vi "fit elliptical orbit to many magnetometer readings.vi"(6 "minimums":T2={"a"=0.0, "b"=-300.0, "theta_axis"=-7.0, "dPhi"=-0.1, "BrV"=-10000.0, "bob tilt"=-0.3, "phi0"=-7.0, "phi_dot"=-1.0, "x0"=-10.0, "y0"=-10.0, "z0"=-200.0}, 7 "maximums":T2={"a"=300.0, "b"=300.0, "theta_axis"=7.0, "dPhi"=0.1, "BrV"=10000.0, "bob tilt"=0.3, "phi0"=7.0, "phi_dot"=1.0, "x0"=10.0, "y0"=10.0, "z0"=200.0}, 8 "t0":fxp<+,48,48>, 9 "omega":dbl, 10 "magnetometer readings":T3[](array[typedef]), 11 "initial parameters":T2) -> (0 "fit field":dbl[](array[numeric]), 1 "measured field":dbl[](array[numeric]), 2 "predicted location":dbl[][](array[numeric]), 3 "fit parameters":T2, 4 "initial field prediction":dbl[](array[numeric]), 5 "initial predicted location":dbl[][](array[numeric]))   [LabVIEW 2017]
uses:
  typedefs/orbit parameters full.ctl
  typedefs/magnetomter reading set.ctl
  typedefs/orbit magnetic field data.ctl
  <vilib>/gmath/NumericalOptimization/Nonlinear Curve Fit TRDL bound.vi
  <vilib>/gmath/NI_Gmath.lvlib
panel:
  out "number of function calls":i32
  out "residue":dbl
  out "initial deriv nan":bool
  out "initial guess nan":bool
  out "XY Graph":T1(graph)
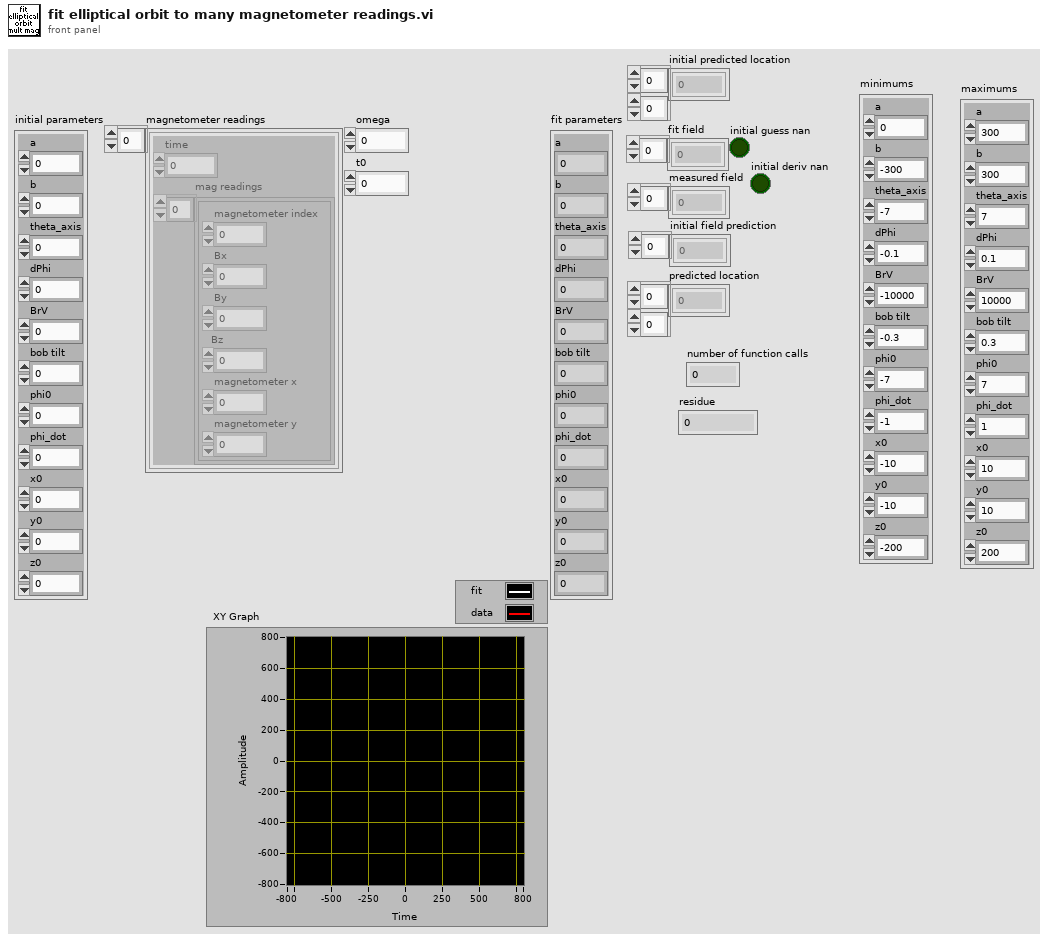
[diagram p1: front panel]
types:
  T1 = cluster{"sensor0 measured":dbl[], "sensor0 measured":dbl[]}[]
  T2 = typedef "orbit parameters full.ctl" = cluster{"a":dbl, "b":dbl, "theta_axis":dbl, "dPhi":dbl, "BrV":dbl, "bob tilt":dbl, "phi0":dbl, "phi_dot":dbl, "x0":dbl, "y0":dbl, "z0":dbl}
  T3 = typedef "magnetomter reading set.ctl" = cluster{"time":fxp<+,48,48>, "mag readings":cluster{"magnetometer index":dbl, "Bx":dbl, "By":dbl, "Bz":dbl, "magnetometer x":dbl, "magnetometer y":dbl}[]}
  T4 = cluster{"parameter minimum":dbl[], "parameter maximum":dbl[]}
  T5 = typedef "orbit magnetic field data.ctl" = cluster{"magnetometer readings":T3[], "L":dbl, "omega":dbl, "t0":fxp<+,48,48>}
  T6 = cluster{"[0]":dbl, "[1]":dbl, "[2]":dbl, "[3]":dbl, "[4]":dbl, "[5]":dbl, "[6]":dbl, "[7]":dbl, "[8]":dbl, "[9]":dbl, "[10]":dbl}
  T7 = cluster{"best fit parameters[0]":dbl, "best fit parameters[1]":dbl, "best fit parameters[2]":dbl, "best fit parameters[3]":dbl, "best fit parameters[4]":dbl, "best fit parameters[5]":dbl, "best fit parameters[6]":dbl, "best fit parameters[7]":dbl, "best fit parameters[8]":dbl, "best fit parameters[9]":dbl, "best fit parameters[10]":dbl}
  T8 = cluster{"sensor0 prediction":dbl[], "sensor0 prediction":dbl[]}
  T9 = cluster{"sensor0 measured":dbl[], "sensor0 measured":dbl[]}
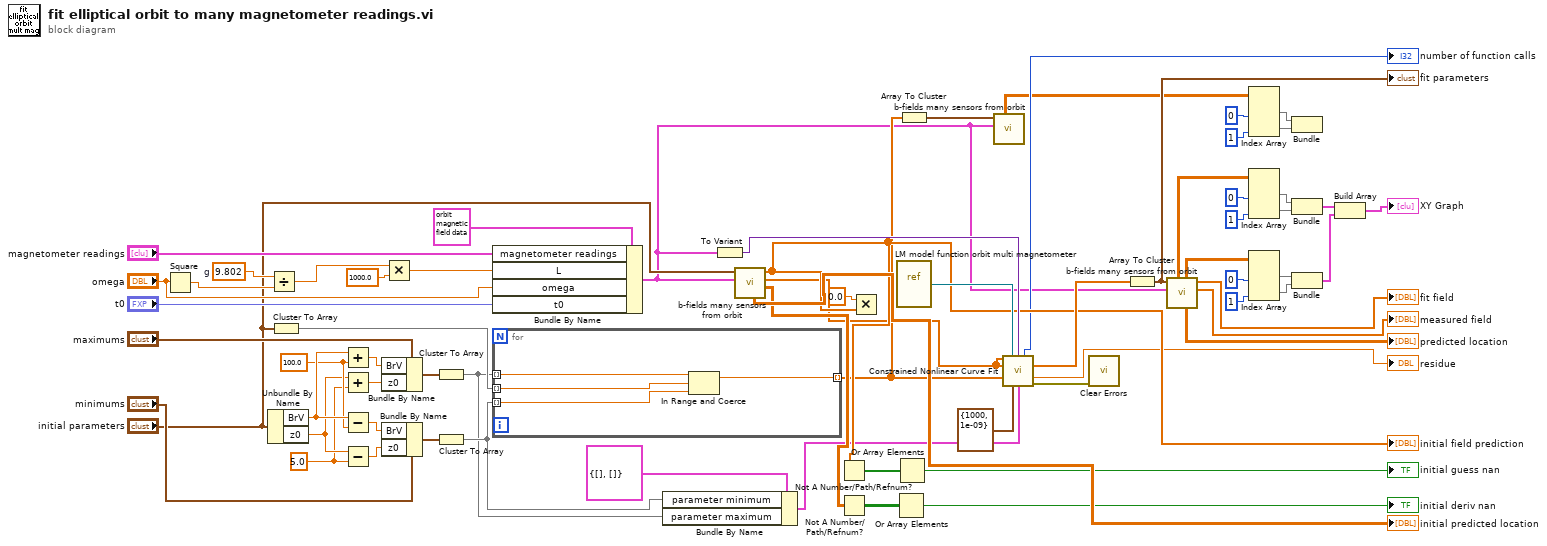
[diagram p0: block diagram]
diagram:
  w20 = 5.0 ("y")
  w23 = 100.0 ("y")
  w62 = 9.802  # g
  n1 = Square(x="omega") -> (x^2=w63:dbl)
  n2 = Unbundle By Name("initial parameters") -> ("BrV"=w24:dbl, "z0"=w21:dbl)
  n3 = Divide(x=w62, y=w63) -> (x/y=w61:dbl)
  n4 = Cluster To Array(cluster="initial parameters") -> (array=w50:dbl[])
  n5 = Add(x=w24, y=w23) -> (x+y=w27:dbl)
  n6 = Add(x=w21, y=w20) -> (x+y=w26:dbl)
  n7 = Subtract(x=w24, y=w23) -> (x-y=w22:dbl)
  n8 = Subtract(x=w21, y=w20) -> (x-y=w19:dbl)
  n9 = Bundle By Name(cluster="maximums", "BrV"=w27, "z0"=w26) -> (w29:T2)
  n10 = Bundle By Name(cluster="minimums", "BrV"=w22, "z0"=w19) -> (w25:T2)
  n11 = Multiply(x=w61, y=1000.0) -> (x*y=w18:dbl)
  n12 = Cluster To Array(cluster=w29) -> (array=w12:dbl[])
  n13 = Cluster To Array(cluster=w25) -> (array=w13:dbl[])
  n14 = Bundle By Name(cluster=T5 {"magnetometer readings"=[], "L"=0.0, "omega"=0.0, "t0"=0.0} ("orbit magnetic field data"), "magnetometer readings"="magnetometer readings", "L"=w18, "omega"="omega", "t0"="t0") -> (w5:T5)
  n15 = for {
    tunnel: w50 -> [w70] mode=indexing
    tunnel: w13 -> [w72] mode=indexing
    tunnel: w12 -> [w71] mode=indexing
    tunnel: [w69] -> w6 mode=indexing
    n16 = In Range and Coerce(upper limit=w71, x=w70, lower limit=w72) -> (coerced(x)=w69:dbl)  [unwired: 1 out]
  }
  n17 = Bundle By Name(cluster=T4 {"parameter minimum"=[], "parameter maximum"=[]} ("parameter bounds"), "parameter minimum"=w13, "parameter maximum"=w12) -> (w11:T4)
  n18 = To Variant(anything=w5) -> (Variant=w54:variant)
  n19 = call "b-fields many sensors from orbit.vi"("orbit magnetic field data"=w5, "orbit parameters"="initial parameters") -> ("derivatives"=w32:dbl[][], "measured field"=w2:dbl[], "predicted field"=w35:dbl[], "predicted location"=→"initial predicted location":dbl[][])  [unwired: 4 in, 2 out]
  "initial field prediction" <- w35
  n20 = Not A Number/Path/Refnum?(number/path/refnum=w35) -> (NaN/Path/Refnum?=w34:bool[])
  n21 = Not A Number/Path/Refnum?(number/path/refnum=w32) -> (NaN/Path/Refnum?=w31:bool[][])
  n22 = Multiply(x=0.0, y=w35) -> ()  [unwired: 1 out]
  n23 = Or Array Elements(Boolean array=w31) -> (logical OR=→"initial deriv nan":bool)
  n24 = vi-ref "LM model function orbit multi magnetometer.vi"() -> (w68:refnum<vi>)
  n25 = Or Array Elements(Boolean array=w34) -> (logical OR=→"initial guess nan":bool)
  n26 = Array To Cluster(array=w6) -> (cluster=w10:T6)
  n27 = call "b-fields many sensors from orbit.vi"("orbit magnetic field data"=w5, "orbit parameters"=w10) -> ("sensor0 prediction"=w4:dbl[][])  [unwired: 4 in, 5 out]
  n28 = call-poly <vilib>:"Constrained Nonlinear Curve Fit.vi"("Y"=w2, "f(x,a)"=w68, "data"=w54, "X"=w2, "initial parameters"=w6, "termination"=cluster{"max iteration":i32, "tolerance":dbl} {"max iteration"=1000, "tolerance"=1e-09}, "parameter bounds"=w11) -> ("number of function calls"=→"number of function calls":i32, "best fit parameters"=w57:dbl[], "residue"=→"residue":dbl, "error out"=w49:errorcluster)  [unwired: 3 in, 2 out]
  n29 = call <vilib>:"Clear Errors.vi"("error in (no error)"=w49) -> ()  [unwired: 5 in, 2 out]
  n30 = Array To Cluster(array=w57) -> (cluster=w55:T7)
  "fit parameters" <- w55
  n31 = call "b-fields many sensors from orbit.vi"("orbit magnetic field data"=w5, "orbit parameters"=w55) -> ("measured field"=→"measured field":dbl[], "predicted field"=→"fit field":dbl[], "predicted location"=→"predicted location":dbl[][], "sensor0 measured"=w47:dbl[][], "sensor0 prediction"=w48:dbl[][])  [unwired: 4 in, 1 out]
  n32 = Index Array(array=w4, index (col) #1=0 ("index (row)"), index (col) #2=1 ("disabled index (col)")) -> (element #1=w9:dbl[], element #2=w8:dbl[])  [unwired: 2 in]
  n33 = Index Array(array=w48, index (col) #1=0 ("index (row)"), index (col) #2=1 ("index (row)")) -> (element #1=w46:dbl[], element #2=w45:dbl[])  [unwired: 2 in]
  n34 = Index Array(array=w47, index (col) #1=0 ("index (row)"), index (col) #2=1 ("disabled index (col)")) -> (element #1=w44:dbl[], element #2=w43:dbl[])  [unwired: 2 in]
  n35 = Bundle("sensor0 prediction"=w9, "sensor0 prediction"=w8) -> ()  [unwired: 1 in, 1 out]
  n36 = Bundle("sensor0 prediction"=w46, "sensor0 prediction"=w45) -> (w42:T8)  [unwired: 1 in]
  n37 = Bundle("sensor0 measured"=w44, "sensor0 measured"=w43) -> (w41:T9)  [unwired: 1 in]
  n38 = Build Array(w42, w41) -> (→"XY Graph":T1)
